vi "PS Control.vi"() -> ()   [LabVIEW 2020]
panel:
  out "Errors":T1(array[cluster]) {"Numeric 2" format="%.4f"; "Numeric" format="%.4f"}
  out "Power Supply State":T2(ring)
  out "Output Cluster":T3 {"MaxLambdaCurrent [A]" format="%.2f"; "LambdaRates [A/min]" format="%.5e"; "MaxNormalCurrent [A]" format="%.2f"; "StabilitySetting [%]" format="%.2f"; "FieldCurrentRatio [T/A]" format="%.2f"; "SwitchWaitTime [s]" format="%.2f"; "SwitchHtrCurrent [mA]" format="%.2f"; "TrainRates [A/min]" format="%.5e"; "NormalRates [A/min]" format="%.5e"; "Breakpts [A]" format="%.5e"}
  in  "Local Enable":bool
  in  "Lambda Mode":bool
  in  "Training Mode":bool
  out "Lambda":bool
  out "Train":bool
  out "Persistent Field":dbl format="%.4f"
  out "Persistence Status":string
  out "Persistent":bool
  in  "Return from persistence":bool
  in  "Make Persistent":bool
  in  "Ramp to Zero":bool
  in  "Hold":bool
  in  "Ramp to Setpoint":bool
  in  "Slew Rate [T/min]":dbl min=0.0 max=5.0 step=0.1 format="%.5f"
  in  "Setpoint [T]":dbl format="%.5f"
  out "Magnet \nVoltage":dbl format="%.2f"
  out "Field [T]":dbl format="%.4f"
  out "Switch Heater Error":bool
  out "Switch heater \nconfirmed":bool
  out "Switch Heater":bool
  in  "VISA session":refnum<visa-resource-name>="GPIB0::22::INSTR"
  in  "stop":bool
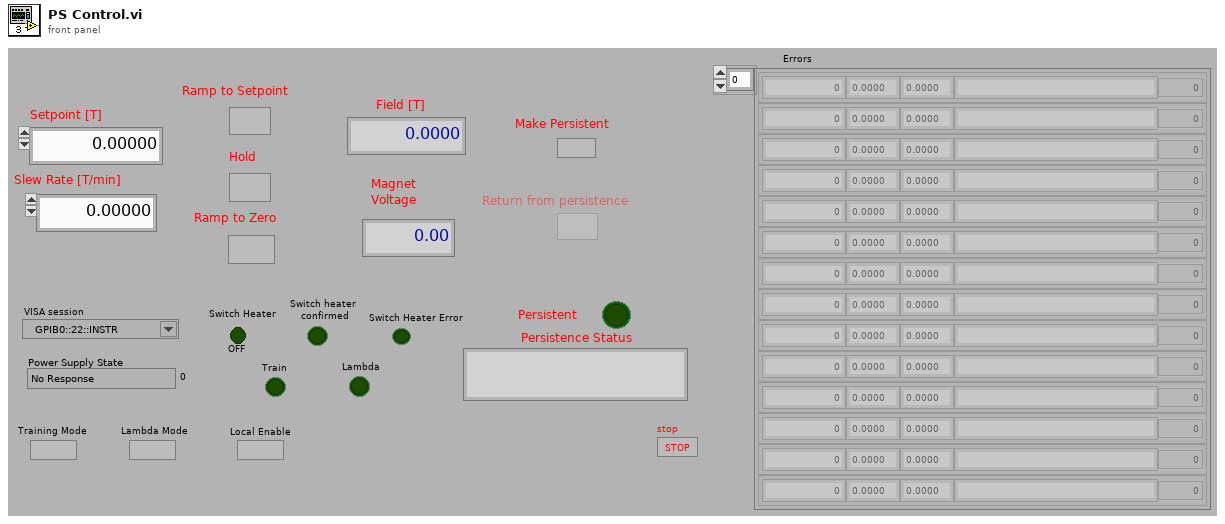
[diagram p1: front panel]
types:
  T1 = cluster{"Index 2":i32, "Numeric":dbl, "Numeric 2":dbl, "String":string, "Read ÆTime(ms)":u32}[]
  T2 = enum16{"No Response", "Ramping to programmed field ", "Holding at programmed field", "Paused", "Ramp Manual Up", "Ramp Manual Down", "Ramping to Zero", "QUENCH", "Heating Persistence Switch", "At Zero Current"}
  T3 = cluster{"Breakpts [A]":dbl[], "NormalRates [A/min]":dbl[], "TrainRates [A/min]":dbl[], "SwitchHtrCurrent [mA]":dbl, "SwitchWaitTime [s]":dbl, "FieldCurrentRatio [T/A]":dbl, "StabilitySetting [%]":dbl, "MaxNormalCurrent [A]":dbl, "Magnet ID":string, "LambdaRates [A/min]":dbl[], "MaxLambdaCurrent [A]":dbl}
  T4 = enum16{"Normal", "Train", "Lambda", "Train & Lambda"}
  T5 = enum8{"Enabled", "Disabled", "Disabled and Grayed Out"}
  T6 = cluster{i32, "Persistent Field":dbl, "Persistent Field":dbl, "String Response":string, "Read ∆ Time":dbl}
  T7 = cluster{"Index 2":i32, "Persistent Field":dbl, "Persistent Field":dbl, "String Response":string, "Read ∆ Time":dbl}[]
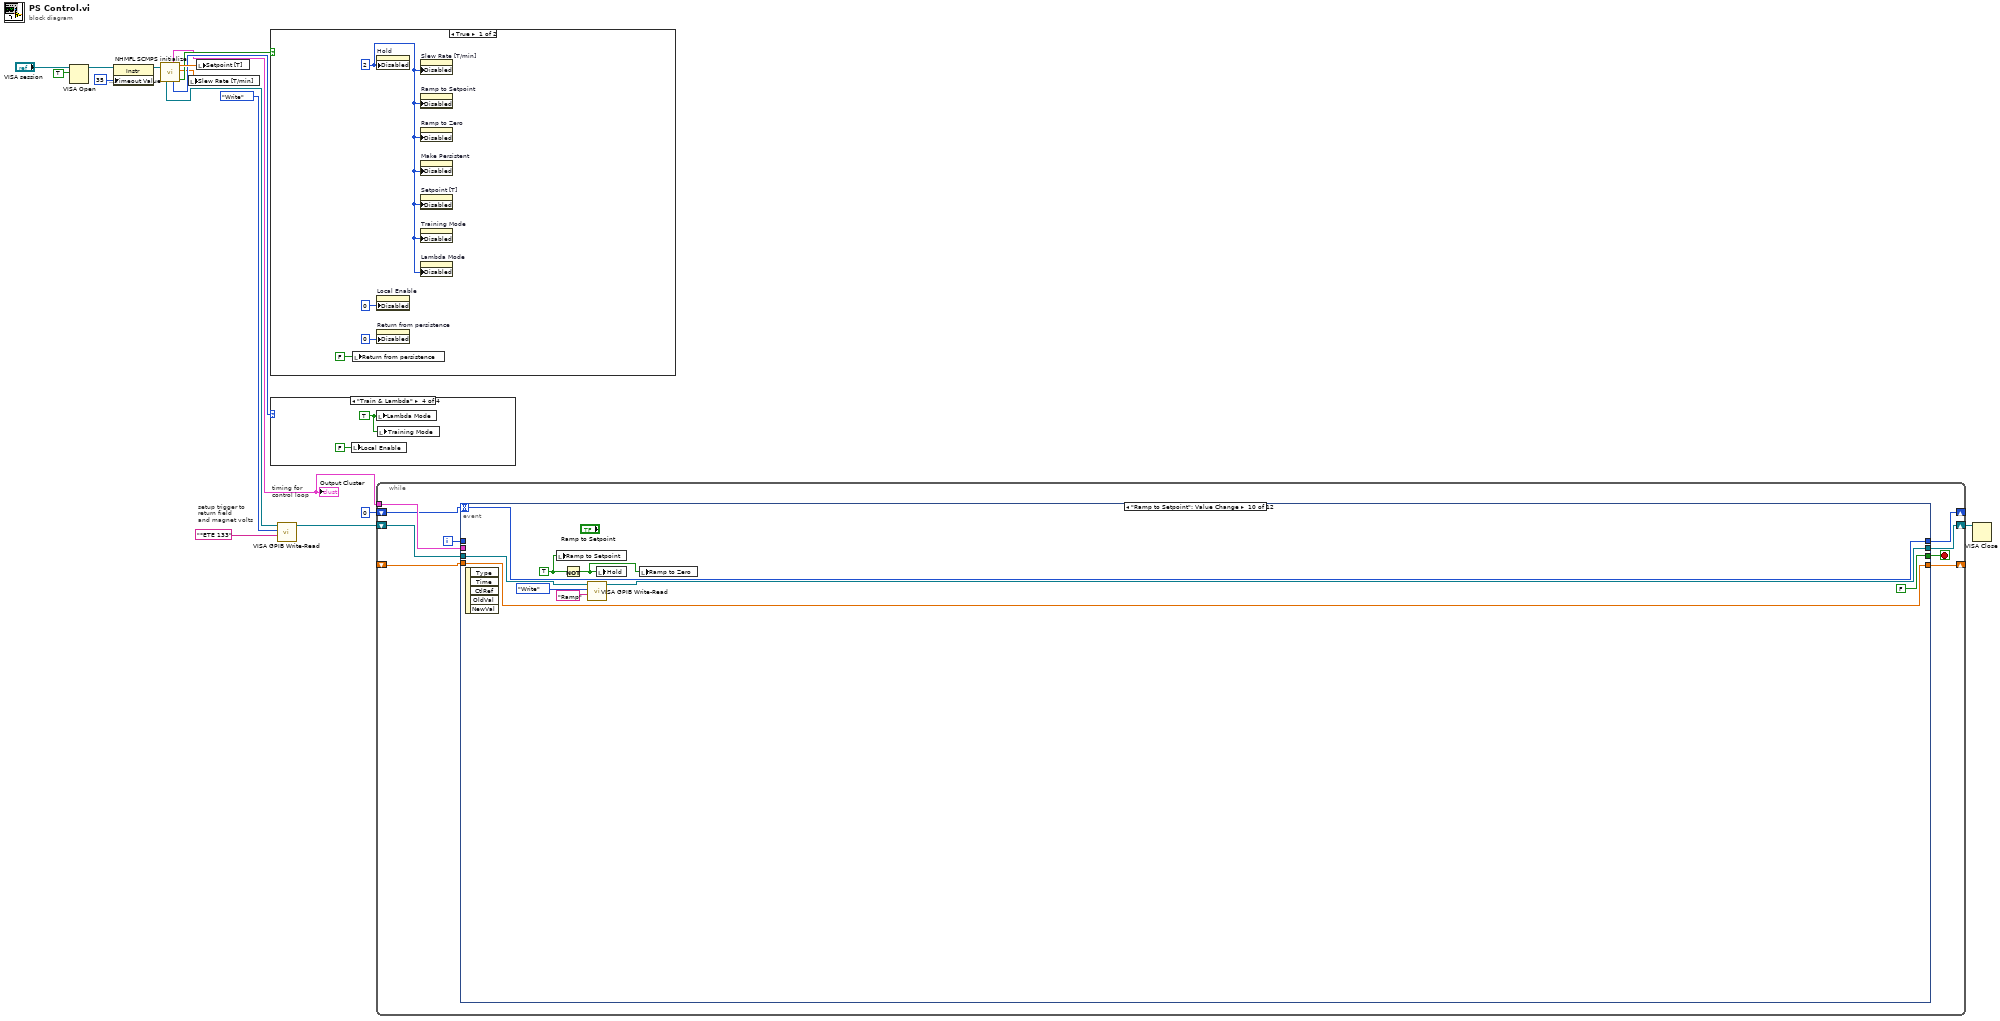
[diagram p0: block diagram]
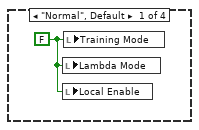
[diagram p2: hidden frame]
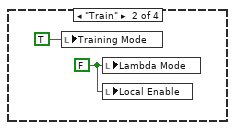
[diagram p3: hidden frame]
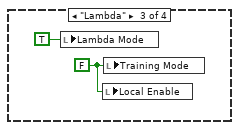
[diagram p4: hidden frame]
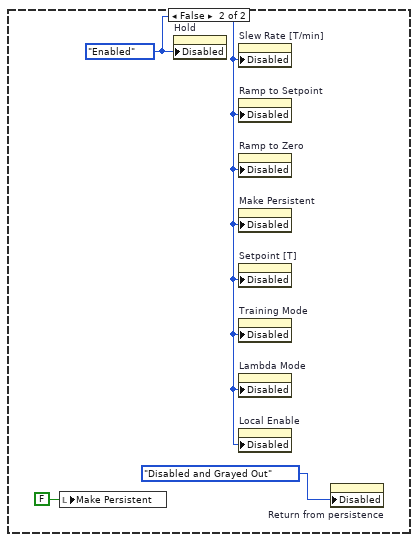
[diagram p5: hidden frame]
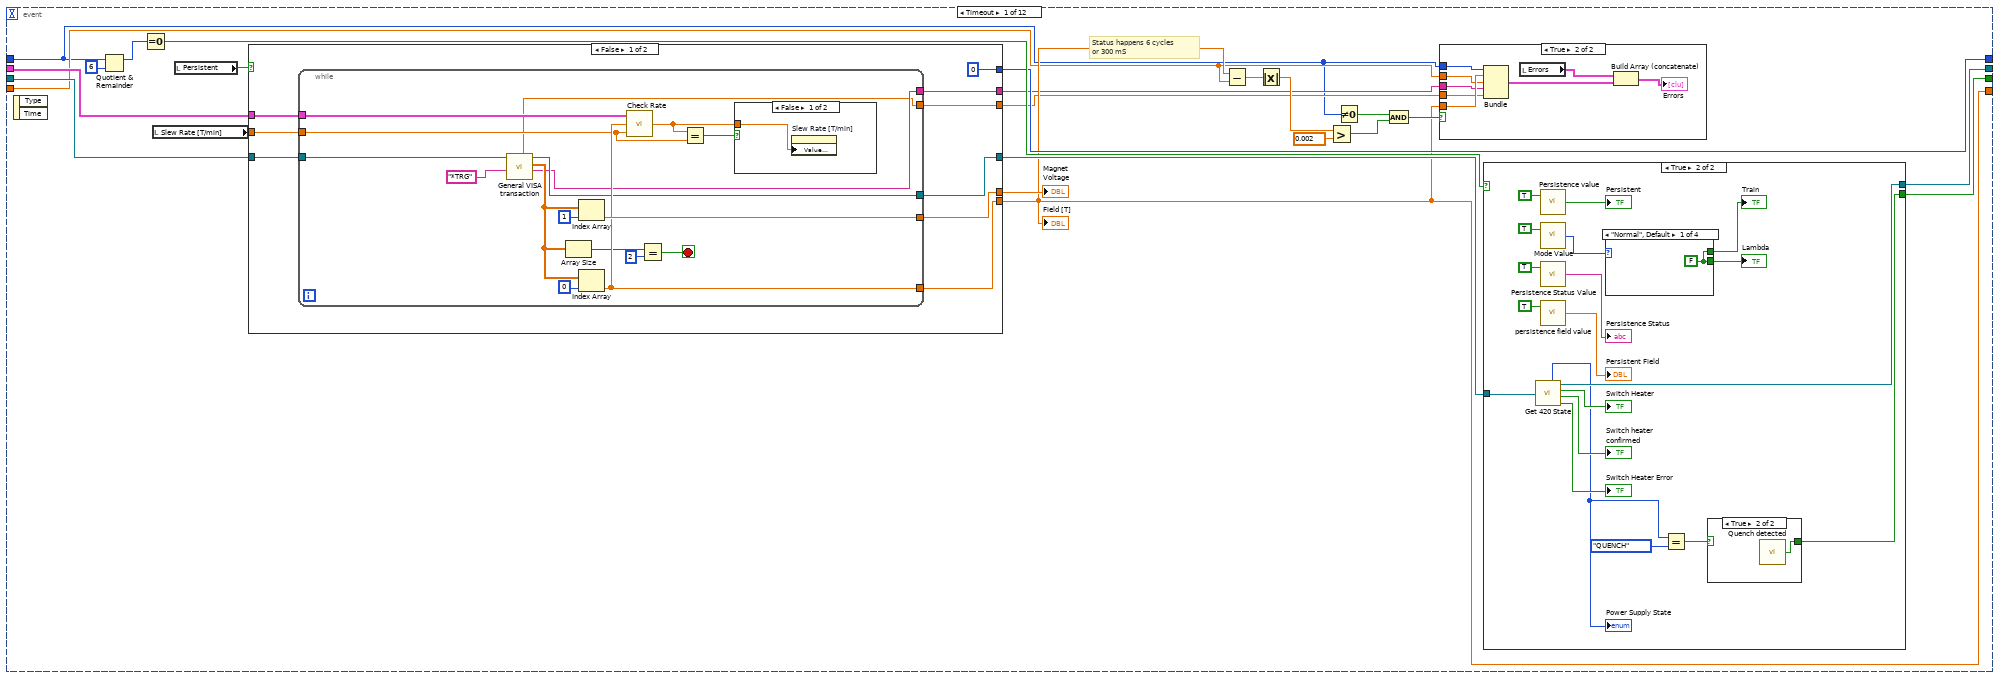
[diagram p6: hidden frame]
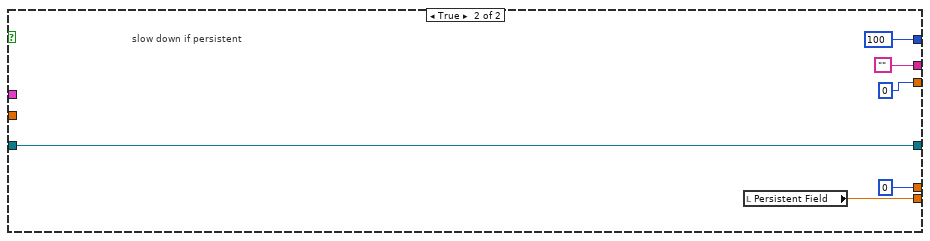
[diagram p9: hidden frame]
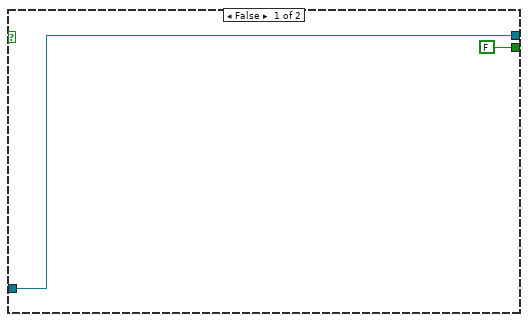
[diagram p10: hidden frame]
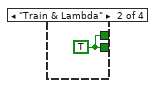
[diagram p12: hidden frame]
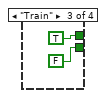
[diagram p13: hidden frame]
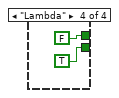
[diagram p14: hidden frame]
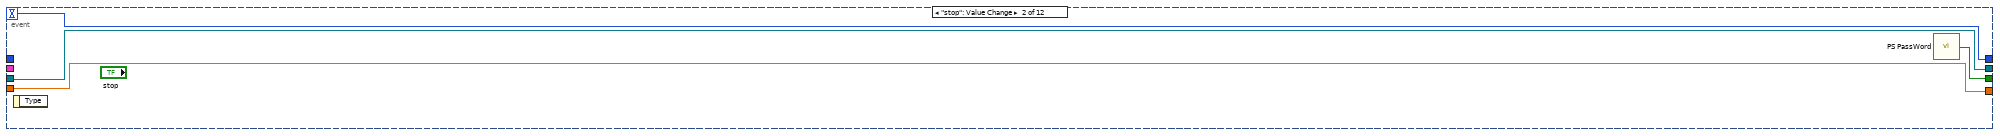
[diagram p15: hidden frame]
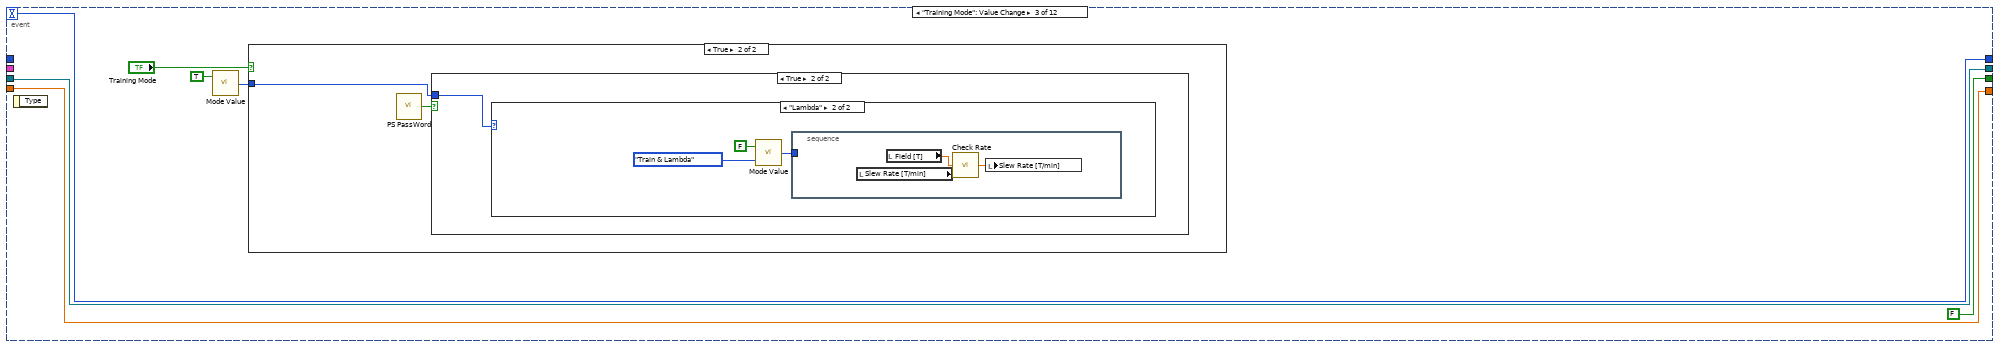
[diagram p16: hidden frame]
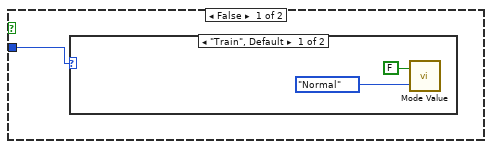
[diagram p17: hidden frame]
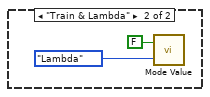
[diagram p18: hidden frame]
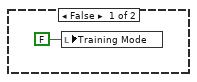
[diagram p19: hidden frame]
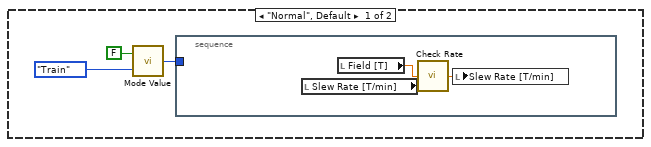
[diagram p20: hidden frame]
diagram:
  # "timing for \ncontrol loop"
  # "setup trigger to \nreturn field\nand magnet volts"
  n1 = VISA Open(duplicate session (F)=TRUE, VISA resource name="VISA session") -> (VISA resource name=w3:refnum<visa-resource-name>)  [unwired: 3 in, 1 out]
  n2 = property class="Instr"(reference=w3, "General Settings:Timeout Value"=u32 35) -> (reference out=w7:refnum<visa-resource-name>)  [unwired: 1 in, 1 out]
  n3 = call "NHMFL SCMPS initialize.vi"("VISA session"=w7) -> ("dup VISA session"=w5:refnum<visa-resource-name>, "Output Cluster"=w6:T3, "Mode Out"=w11:T4, "Programmed Field"=w14:dbl, "Ramp Rate"=w10:dbl, "Persistent"=w12:bool)  [unwired: 1 out]
  "Output Cluster" <- w6
  n4 = local write "Slew Rate [T/min]"(w10) -> ()
  n5 = local write "Setpoint [T]"(w14) -> ()
  n6 = case shown="True" w12 {
    frame True {
      w18 = 2
      n7 = local write "Return from persistence"(FALSE ("Return from persistence")) -> ()
      n8 = property on="Hold" class="Bool (strict)"("Disabled"=w18) -> ()  [unwired: 2 in, 2 out]
      n9 = property on="Local Enable" class="Bool (strict)"("Disabled"=u8 0) -> ()  [unwired: 2 in, 2 out]
      n10 = property on="Return from persistence" class="Bool (strict)"("Disabled"=u8 0) -> ()  [unwired: 2 in, 2 out]
      n11 = property on="Slew Rate [T/min]" class="DigNum (strict)"("Disabled"=w18) -> ()  [unwired: 2 in, 2 out]
      n12 = property on="Ramp to Setpoint" class="Bool (strict)"("Disabled"=w18) -> ()  [unwired: 2 in, 2 out]
      n13 = property on="Ramp to Zero" class="Bool (strict)"("Disabled"=w18) -> ()  [unwired: 2 in, 2 out]
      n14 = property on="Make Persistent" class="Bool (strict)"("Disabled"=w18) -> ()  [unwired: 2 in, 2 out]
      n15 = property on="Setpoint [T]" class="DigNum (strict)"("Disabled"=w18) -> ()  [unwired: 2 in, 2 out]
      n16 = property on="Training Mode" class="Bool (strict)"("Disabled"=w18) -> ()  [unwired: 2 in, 2 out]
      n17 = property on="Lambda Mode" class="Bool (strict)"("Disabled"=w18) -> ()  [unwired: 2 in, 2 out]
    }
    frame False {
      w22 = T5."Enabled" ("Disabled")
      n18 = local write "Make Persistent"(FALSE ("Return from persistence")) -> ()
      n19 = property on="Hold" class="Bool (strict)"("Disabled"=w22) -> ()  [unwired: 2 in, 2 out]
      n20 = property on="Slew Rate [T/min]" class="DigNum (strict)"("Disabled"=w22) -> ()  [unwired: 2 in, 2 out]
      n21 = property on="Ramp to Setpoint" class="Bool (strict)"("Disabled"=w22) -> ()  [unwired: 2 in, 2 out]
      n22 = property on="Ramp to Zero" class="Bool (strict)"("Disabled"=w22) -> ()  [unwired: 2 in, 2 out]
      n23 = property on="Make Persistent" class="Bool (strict)"("Disabled"=w22) -> ()  [unwired: 2 in, 2 out]
      n24 = property on="Setpoint [T]" class="DigNum (strict)"("Disabled"=w22) -> ()  [unwired: 2 in, 2 out]
      n25 = property on="Training Mode" class="Bool (strict)"("Disabled"=w22) -> ()  [unwired: 2 in, 2 out]
      n26 = property on="Lambda Mode" class="Bool (strict)"("Disabled"=w22) -> ()  [unwired: 2 in, 2 out]
      n27 = property on="Local Enable" class="Bool (strict)"("Disabled"=w22) -> ()  [unwired: 2 in, 2 out]
      n28 = property on="Return from persistence" class="Bool (strict)"("Disabled"=T5."Disabled and Grayed Out") -> ()  [unwired: 2 in, 2 out]
    }
  }
  n29 = case shown="\"Train & Lambda\"" w11 {
    frame "Normal", Default {
      w24 = FALSE ("Training Mode")
      n30 = local write "Lambda Mode"(w24) -> ()
      n31 = local write "Local Enable"(w24) -> ()
      n32 = local write "Training Mode"(w24) -> ()
    }
    frame "Train" {
      w26 = FALSE
      n33 = local write "Training Mode"(TRUE) -> ()
      n34 = local write "Lambda Mode"(w26) -> ()
      n35 = local write "Local Enable"(w26) -> ()
    }
    frame "Lambda" {
      w27 = FALSE
      n36 = local write "Lambda Mode"(TRUE) -> ()
      n37 = local write "Local Enable"(w27) -> ()
      n38 = local write "Training Mode"(w27) -> ()
    }
    frame "Train & Lambda" {
      w29 = TRUE
      n39 = local write "Local Enable"(FALSE) -> ()
      n40 = local write "Lambda Mode"(w29) -> ()
      n41 = local write "Training Mode"(w29) -> ()
    }
  }
  n42 = call "VISA GPIB Write-Read.vi"("Command"="*ETE 133" ("Command String"), "Action"=enum16{"Write", "Read", "Write & Read"}."Write", "VISA resource name"=w5) -> ("dup VISA Session"=w4:refnum<visa-resource-name>)  [unwired: 5 in, 3 out]
  n43 = while {
    tunnel: w6 -> [w38]
    shift-right: [w35] -> w1
    shift-left: w4 -> [w39]
    shift-right: [w33] -> _
    shift-left: 0 ("y") -> [w34]
    shift-right: [w32] -> _
    shift-left: _ -> [w31]
    i -> [w37]
    stop <- w36 stop-if-true
    n44 = event shown="[9] \"Ramp to Setpoint\": Value Change" {
      selector: _ -> [_ _ _ _ _ _ _ _ _ _ _ _]
      dyn-events: _ -> [_ _ _ _ _ _ _ _ _ _ _ _]
      timeout: w34 -> [_ w134 w138 w166 w194 w221 w274 w286 w316 w328 w337 w346]
      tunnel: w39 -> [w57 w135 w139 w167 w199 w231 w275 w291 w325 w335 w342 w351]
      tunnel: [w55 w136 FALSE ("Password Correct") FALSE ("Password Correct") FALSE ("Password Correct") FALSE ("Password Correct") FALSE ("Password Correct") FALSE ("Password Correct") FALSE ("Password Correct") FALSE ("Password Correct") FALSE ("Password Correct") FALSE ("Password Correct")] -> w36
      tunnel: w38 -> [w54 _ _ _ w198 w225 _ _ w318 _ _ _]
      tunnel: w37 -> [w40 _ _ _ _ _ _ _ _ _ _ _]
      tunnel: [w53 w135 w139 w167 w195 w222 w275 w290 w317 w329 w338 w347] -> w35
      tunnel: [w52 w134 w138 w166 w194 w221 w274 w286 w316 w328 w337 w346] -> w33
      tunnel: [w45 w133 w137 w165 w193 w220 w273 w285 w315 w327 w336 w345] -> w32
      tunnel: w31 -> [w43 w133 w137 w165 w193 w220 w273 w285 w315 w327 w336 w345]
      event Timeout {
        # "Status happens 6 cycles\nor 300 mS"
        n45 = event-data() -> ()  [unwired: 1 in, 2 out]
        n46 = Quotient & Remainder(x=w40, y=6) -> (x-y*floor(x/y)=w44:i32)  [unwired: 1 out]
        n47 = Equal To 0?(x=w44) -> (x = 0?=w61:bool)
        n48 = local read "Slew Rate [T/min]"() -> (w60:dbl)
        n49 = local read "Persistent"() -> (w59:bool)
        n50 = case shown="False" w59 {
          tunnel: w57 -> [w79 w101]
          tunnel: [w77 w103] -> w45
          tunnel: [w78 0] -> w58
          tunnel: w54 -> [w76 _]
          tunnel: w60 -> [w75 _]
          tunnel: [w74 w101] -> w56
          tunnel: [0 ("y") 100 ("y")] -> w52
          tunnel: [w72 "" ("String Response")] -> w42
          tunnel: [w71 u32 0 ("Read ÆTime")] -> w41
          frame False {
            n51 = while {
              tunnel: w79 -> [w83]
              tunnel: [w96] -> w78
              tunnel: [w95] -> w77
              tunnel: w76 -> [w94]
              tunnel: w75 -> [w86]
              tunnel: [w82] -> w74
              tunnel: [w81] -> w72
              tunnel: [w80] -> w71
              stop <- w87 stop-if-true
              n52 = call "General VISA transaction.vi"("Command String"="*TRG", "VISA Session"=w83) -> ("String Resonse"=w81:string, "Measurement"=w90:dbl[], "dup VISA Session"=w82:refnum<visa-resource-name>, "Read ∆ Time"=w80:dbl)  [unwired: 4 in, 2 out]
              n53 = Array Size(array=w90) -> (size(s)=w89:i32)
              n54 = Index Array(array=w90, index=1) -> (element=w96:dbl)
              n55 = Index Array(array=w90, index=0) -> (element=w95:dbl)
              n56 = call "Check Rate.vi"("Rate"=w86, "Field"=w95, "input cluster"=w94) -> ("Checked Rate"=w84:dbl)
              n57 = Equal?(x=w89, y=2) -> (x = y?=w87:bool)
              n58 = Equal?(x=w84, y=w86) -> (x = y?=w85:bool)
              n59 = case shown="False" w85 {
                tunnel: w84 -> [w97 _]
                frame False {
                  n60 = property on="Slew Rate [T/min]" class="DigNum (strict)"("Value (Signaling)"=w97) -> ()  [unwired: 2 in, 2 out]
                }
                frame True {
                }
              }
            }
          }
          frame True {
            # "slow down if persistent"
            n61 = local read "Persistent Field"() -> (w103:dbl)
          }
        }
        "Field [T]" <- w45
        "Magnet \nVoltage" <- w58
        n62 = Subtract(x=w45, y=w43) -> (x-y=w51:dbl)
        n63 = Absolute Value(x=w51) -> (abs(x)=w50:dbl)
        n64 = Greater?(x=w50, y=0.002) -> (0:w49:bool)
        n65 = Not Equal To 0?(x=w40) -> (x != 0?=w48:bool)
        n66 = And(x=w48, y=w49) -> (x .and. y?=w46:bool)
        n67 = case shown="True" w46 {
          tunnel: w45 -> [_ w70]
          tunnel: w43 -> [_ w69]
          tunnel: w42 -> [_ w67]
          tunnel: w40 -> [_ w64]
          tunnel: w41 -> [_ w63]
          frame False {
          }
          frame True {
            n68 = Bundle(w64, "Persistent Field"=w70, "Persistent Field"=w69, "String Response"=w67, "Read ∆ Time"=w63) -> (w66:T6)  [unwired: 1 in]
            n69 = local read "Errors"() -> (w68:T1)
            n70 = Build Array (concatenate)(w68, w66) -> (→"Errors":T7)
          }
        }
        n71 = case shown="True" w61 {
          tunnel: w56 -> [w104 w108]
          tunnel: [FALSE w109] -> w55
          tunnel: [w104 w107] -> w53
          frame False {
          }
          frame True {
            n72 = call "Get 420 State.vi"("VISA session"=w108) -> ("State"=w106:T2, "dup VISA session"=w107:refnum<visa-resource-name>, "Switch Heater"=→"Switch Heater":bool, "Switch heater \nconfirmed"=→"Switch heater \nconfirmed":bool, "Switch Heater Error"=→"Switch Heater Error":bool)  [unwired: 1 out]
            "Power Supply State" <- w106
            n73 = call "Persistence value.vi"("Read/Write this vi"=TRUE) -> ("Persistence Out"=→"Persistent":bool)  [unwired: 1 in]
            n74 = call "Mode Value.vi"("Read/Write this vi"=TRUE) -> ("Mode Out"=w120:T4)  [unwired: 1 in]
            n75 = call "Persistence Status Value.vi"("Read/Write this vi"=TRUE) -> ("Persistence Status Out"=→"Persistence Status":string)  [unwired: 1 in]
            n76 = call "persistence field value.vi"("Read/Write this vi"=TRUE) -> ("Persistent Field Out"=→"Persistent Field":dbl)  [unwired: 1 in]
            n77 = case shown="\"Normal\", Default" w120 {
              tunnel: [w127 w128 TRUE FALSE] -> w121
              tunnel: [w127 w128 FALSE TRUE] -> w122
              frame "Normal", Default {
                w127 = FALSE
              }
              frame "Train & Lambda" {
                w128 = TRUE
              }
              frame "Train" {
              }
              frame "Lambda" {
              }
            }
            "Train" <- w121
            "Lambda" <- w122
            n78 = Equal?(x=w106, y=T2."QUENCH" ("x")) -> (x = y?=w111:bool)
            n79 = case shown="True" w111 {
              selector: w111 -> [w125 _]
              tunnel: [w125 w126] -> w109
              frame False {
              }
              frame True {
                n80 = call "Quench detected.vi"() -> ("Stop"=w126:bool)
              }
            }
          }
        }
      }
      event "stop": Value Change {
        n81 = event-data() -> ()  [unwired: 1 in, 1 out]
        n82 = call "PS PassWord.vi"() -> ("Password Correct"=w136:bool)  [unwired: 2 in]
      }
      event "Training Mode": Value Change {
        n83 = event-data() -> ()  [unwired: 1 in, 1 out]
        n84 = call "Mode Value.vi"("Read/Write this vi"=TRUE) -> ("Mode Out"=w141:T4)  [unwired: 1 in]
        n85 = case shown="True" "Training Mode" {
          tunnel: w141 -> [w144 w149]
          frame False {
            n86 = case shown="\"Train\", Default" w144 {
              frame "Train", Default {
                n87 = call "Mode Value.vi"("Mode In"=T4."Normal", "Read/Write this vi"=FALSE) -> ()  [unwired: 1 out]
              }
              frame "Train & Lambda" {
                n88 = call "Mode Value.vi"("Mode In"=T4."Lambda", "Read/Write this vi"=FALSE) -> ()  [unwired: 1 out]
              }
            }
          }
          frame True {
            n89 = call "PS PassWord.vi"() -> ("Password Correct"=w150:bool)  [unwired: 2 in]
            n90 = case shown="True" w150 {
              tunnel: w149 -> [_ w152]
              frame False {
                n91 = local write "Training Mode"(FALSE ("Train")) -> ()
              }
              frame True {
                n92 = case shown="\"Lambda\"" w152 {
                  frame "Normal", Default {
                    n93 = call "Mode Value.vi"("Mode In"=T4."Train", "Read/Write this vi"=FALSE) -> ("Mode Out"=w153:T4)
                    n94 = stacked-sequence {
                      tunnel: w153 -> [_]
                      frame #0 {
                        n95 = local read "Slew Rate [T/min]"() -> (w158:dbl)
                        n96 = local read "Field [T]"() -> (w157:dbl)
                        n97 = call "Check Rate.vi"("Rate"=w158, "Field"=w157) -> ("Checked Rate"=w156:dbl)  [unwired: 1 in]
                        n98 = local write "Slew Rate [T/min]"(w156) -> ()
                      }
                    }
                  }
                  frame "Lambda" {
                    n99 = call "Mode Value.vi"("Mode In"=T4."Train & Lambda", "Read/Write this vi"=FALSE) -> ("Mode Out"=w159:T4)
                    n100 = stacked-sequence {
                      tunnel: w159 -> [_]
                      frame #0 {
                        n101 = local read "Slew Rate [T/min]"() -> (w164:dbl)
                        n102 = local read "Field [T]"() -> (w163:dbl)
                        n103 = call "Check Rate.vi"("Rate"=w164, "Field"=w163) -> ("Checked Rate"=w162:dbl)  [unwired: 1 in]
                        n104 = local write "Slew Rate [T/min]"(w162) -> ()
                      }
                    }
                  }
                }
              }
            }
          }
        }
      }
      event "Lambda Mode": Value Change {
        n105 = event-data() -> ()  [unwired: 1 in, 1 out]
        n106 = call "Mode Value.vi"("Read/Write this vi"=TRUE) -> ("Mode Out"=w169:T4)  [unwired: 1 in]
        n107 = case shown="True" "Lambda Mode" {
          tunnel: w169 -> [w172 w177]
          frame False {
            n108 = case shown="\"Lambda\", Default" w172 {
              frame "Lambda", Default {
                n109 = call "Mode Value.vi"("Mode In"=T4."Normal", "Read/Write this vi"=FALSE) -> ()  [unwired: 1 out]
              }
              frame "Train & Lambda" {
                n110 = call "Mode Value.vi"("Mode In"=T4."Train", "Read/Write this vi"=FALSE) -> ()  [unwired: 1 out]
              }
            }
          }
          frame True {
            n111 = call "PS PassWord.vi"() -> ("Password Correct"=w178:bool)  [unwired: 2 in]
            n112 = case shown="True" w178 {
              tunnel: w177 -> [_ w180]
              frame False {
                n113 = local write "Lambda Mode"(FALSE) -> ()
              }
              frame True {
                n114 = case shown="\"Train\"" w180 {
                  frame "Train" {
                    n115 = call "Mode Value.vi"("Mode In"=T4."Train & Lambda", "Read/Write this vi"=FALSE) -> ("Mode Out"=w181:T4)
                    n116 = stacked-sequence {
                      tunnel: w181 -> [_]
                      frame #0 {
                        n117 = local read "Slew Rate [T/min]"() -> (w186:dbl)
                        n118 = local read "Field [T]"() -> (w185:dbl)
                        n119 = call "Check Rate.vi"("Rate"=w186, "Field"=w185) -> ("Checked Rate"=w184:dbl)  [unwired: 1 in]
                        n120 = local write "Slew Rate [T/min]"(w184) -> ()
                      }
                    }
                  }
                  frame "Normal", Default {
                    n121 = call "Mode Value.vi"("Mode In"=T4."Lambda", "Read/Write this vi"=FALSE) -> ("Mode Out"=w187:T4)
                    n122 = stacked-sequence {
                      tunnel: w187 -> [_]
                      frame #0 {
                        n123 = local read "Slew Rate [T/min]"() -> (w192:dbl)
                        n124 = local read "Field [T]"() -> (w191:dbl)
                        n125 = call "Check Rate.vi"("Rate"=w192, "Field"=w191) -> ("Checked Rate"=w190:dbl)  [unwired: 1 in]
                        n126 = local write "Slew Rate [T/min]"(w190) -> ()
                      }
                    }
                  }
                }
              }
            }
          }
        }
      }
      event "Local Enable": Value Change {
        n127 = event-data() -> ("NewVal"=w197:bool)  [unwired: 1 in]
        n128 = case shown="True" w197 {
          tunnel: w199 -> [w202 w210]
          tunnel: w198 -> [_ w209]
          tunnel: [w200 w207] -> w195
          frame False {
            n129 = call "VISA GPIB Write-Read.vi"("Command"="SYST:REM" ("Command String"), "Action"=enum16{"Write", "Read", "Write & Read"}."Write", "VISA resource name"=w202) -> ("dup VISA Session"=w201:refnum<visa-resource-name>)  [unwired: 5 in, 3 out]
            n130 = stacked-sequence {
              tunnel: w201 -> [w205]
              tunnel: [w205] -> w200
              frame #0 {
                n131 = local write "Local Enable"(FALSE ("Local Enable")) -> ()
              }
            }
          }
          frame True {
            n132 = call "PS PassWord.vi"() -> ("Password Correct"=w208:bool)  [unwired: 2 in]
            n133 = case shown="True" w208 {
              tunnel: w210 -> [w211 w215]
              tunnel: w209 -> [_ _]
              tunnel: [w211 w213] -> w207
              frame False {
                n134 = local write "Local Enable"(FALSE) -> ()
              }
              frame True {
                n135 = call "VISA GPIB Write-Read.vi"("Command"="SYST:LOC" ("Command String"), "Action"=enum16{"Write", "Read", "Write & Read"}."Write", "VISA resource name"=w215) -> ("dup VISA Session"=w214:refnum<visa-resource-name>)  [unwired: 5 in, 3 out]
                n136 = stacked-sequence {
                  tunnel: w214 -> [w218]
                  tunnel: [w218] -> w213
                  frame #0 {
                    n137 = local write "Local Enable"(TRUE) -> ()
                  }
                }
              }
            }
          }
        }
      }
      event "Setpoint [T]": Value Change {
        n138 = event-data() -> ()  [unwired: 1 in, 5 out]
        n139 = call "Mode Value.vi"("Read/Write this vi"=TRUE) -> ("Mode Out"=w227:T4)  [unwired: 1 in]
        n140 = case shown="\"Train & Lambda\"" w227 {
          tunnel: "Setpoint [T]" -> [w235 w244 w254 w264]
          tunnel: w225 -> [w242 w252 w262 w272]
          tunnel: [w234 w246 w256 w266] -> w224
          frame "Normal", Default {
            n141 = Unbundle By Name(w242) -> ("MaxNormalCurrent [A]"=w240:dbl, "FieldCurrentRatio [T/A]"=w239:dbl)
            n142 = Multiply(x=w240, y=w239) -> (x*y=w241:dbl)
            n143 = Absolute Value(x=w235) -> (abs(x)=w238:dbl)
            n144 = In Range and Coerce(upper limit=w241, x=w238, lower limit=0.0) -> (coerced(x)=w236:dbl)  [unwired: 1 out]
            n145 = Sign(1:w235) -> (0:w233:dbl)
            n146 = Multiply(x=w236, y=w233) -> (x*y=w234:dbl)
          }
          frame "Train" {
            n147 = Unbundle By Name(w252) -> ("MaxNormalCurrent [A]"=w250:dbl, "FieldCurrentRatio [T/A]"=w249:dbl)
            n148 = Multiply(x=w250, y=w249) -> (x*y=w251:dbl)
            n149 = Absolute Value(x=w244) -> (abs(x)=w248:dbl)
            n150 = In Range and Coerce(upper limit=w251, x=w248, lower limit=0.0) -> (coerced(x)=w245:dbl)  [unwired: 1 out]
            n151 = Sign(1:w244) -> (0:w243:dbl)
            n152 = Multiply(x=w245, y=w243) -> (x*y=w246:dbl)
          }
          frame "Lambda" {
            n153 = Unbundle By Name(w262) -> ("MaxLambdaCurrent [A]"=w260:dbl, "FieldCurrentRatio [T/A]"=w259:dbl)
            n154 = Multiply(x=w260, y=w259) -> (x*y=w261:dbl)
            n155 = Absolute Value(x=w254) -> (abs(x)=w258:dbl)
            n156 = In Range and Coerce(upper limit=w261, x=w258, lower limit=0.0) -> (coerced(x)=w255:dbl)  [unwired: 1 out]
            n157 = Sign(1:w254) -> (0:w253:dbl)
            n158 = Multiply(x=w255, y=w253) -> (x*y=w256:dbl)
          }
          frame "Train & Lambda" {
            n159 = Unbundle By Name(w272) -> ("MaxLambdaCurrent [A]"=w270:dbl, "FieldCurrentRatio [T/A]"=w269:dbl)
            n160 = Multiply(x=w270, y=w269) -> (x*y=w271:dbl)
            n161 = Absolute Value(x=w264) -> (abs(x)=w268:dbl)
            n162 = In Range and Coerce(upper limit=w271, x=w268, lower limit=0.0) -> (coerced(x)=w265:dbl)  [unwired: 1 out]
            n163 = Sign(1:w264) -> (0:w263:dbl)
            n164 = Multiply(x=w265, y=w263) -> (x*y=w266:dbl)
          }
        }
        n165 = local write "Setpoint [T]"(w224) -> ()
        n166 = Format Into String(format string="CONF:FIELD:PROG %f" ("Command String"), w224) -> (resulting string=w230:string)  [unwired: 2 in, 1 out]
        n167 = call "VISA GPIB Write-Read.vi"("Command"=w230, "Action"=enum16{"Write", "Read", "Write & Read"}."Write", "VISA resource name"=w231) -> ("dup VISA Session"=w222:refnum<visa-resource-name>)  [unwired: 5 in, 3 out]
      }
      event "Make Persistent": Value Change {
        n168 = event-data() -> ()  [unwired: 1 in, 5 out]
        n169 = flat-sequence {
          tunnel: w275 -> [w278]
          tunnel: [w278] -> w276
          tunnel: w276 -> [w281]
          frame #0 {
            w280 = u8 2 ("Disabled")
            # "Disable controls"
            n170 = property on="Make Persistent" class="Bool (strict)"("Disabled"=w280) -> ()  [unwired: 2 in, 2 out]
            n171 = property on="Return from persistence" class="Bool (strict)"("Disabled"=w280) -> ()  [unwired: 2 in, 2 out]
            n172 = property on="Training Mode" class="Bool (strict)"("Disabled"=w280) -> ()  [unwired: 2 in, 2 out]
            n173 = property on="Lambda Mode" class="Bool (strict)"("Disabled"=w280) -> ()  [unwired: 2 in, 2 out]
            n174 = property on="Local Enable" class="Bool (strict)"("Disabled"=w280) -> ()  [unwired: 2 in, 2 out]
            n175 = property on="Persistence Status" class="Str"("Blinking"=TRUE) -> ()  [unwired: 2 in, 2 out]
            n176 = property on="Hold" class="Bool (strict)"("Disabled"=w280) -> ()  [unwired: 2 in, 2 out]
            n177 = property on="Slew Rate [T/min]" class="DigNum (strict)"("Disabled"=w280) -> ()  [unwired: 2 in, 2 out]
            n178 = property on="Ramp to Setpoint" class="Bool (strict)"("Disabled"=w280) -> ()  [unwired: 2 in, 2 out]
            n179 = property on="Ramp to Zero" class="Bool (strict)"("Disabled"=w280) -> ()  [unwired: 2 in, 2 out]
            n180 = property on="Setpoint [T]" class="DigNum (strict)"("Disabled"=w280) -> ()  [unwired: 2 in, 2 out]
          }
          frame #1 {
            # "make persistent routine"
            n181 = call "NML SCMPS make persistent.vi"("VISA session"=w281) -> ()  [unwired: 1 in, 3 out]
          }
          frame #2 {
            # "enable return from persistence control"
            n182 = local write "Return from persistence"(FALSE ("Return from persistence")) -> ()
            n183 = property on="Persistence Status" class="Str"("Blinking"=FALSE) -> ()  [unwired: 2 in, 2 out]
            n184 = property on="Return from persistence" class="Bool (strict)"("Disabled"=u8 0) -> ()  [unwired: 2 in, 2 out]
          }
        }
      }
      event "Return from persistence": Value Change {
        n185 = event-data() -> ()  [unwired: 1 in, 1 out]
        n186 = flat-sequence {
          tunnel: w291 -> [w294]
          tunnel: [w294] -> w289
          tunnel: w289 -> [w297]
          tunnel: [w296] -> w288
          tunnel: w288 -> [w307]
          tunnel: [w298] -> w287
          tunnel: [w310] -> w290
          tunnel: w287 -> [w310]
          frame #0 {
            w293 = T5."Disabled and Grayed Out" ("Disabled")
            # "disable both controls (others should already be disabled)"
            n187 = property on="Persistence Status" class="Str"("Blinking"=TRUE) -> ()  [unwired: 2 in, 2 out]
            n188 = property on="Make Persistent" class="Bool (strict)"("Disabled"=w293) -> ()  [unwired: 2 in, 2 out]
            n189 = property on="Return from persistence" class="Bool (strict)"("Disabled"=w293) -> ()  [unwired: 2 in, 2 out]
          }
          frame #1 {
            # "run return from persistence vi"
            n190 = call "NML SCMPS unpersistence.vi"("VISA session"=w297) -> ("dup VISA session"=w296:refnum<visa-resource-name>)  [unwired: 2 in, 2 out]
          }
          frame #2 {
            # "enable all controls except return from persistence \nand change rate back to normal"
            n191 = local read "Slew Rate [T/min]"() -> (w305:dbl)
            n192 = local read "Setpoint [T]"() -> (w300:dbl)
            n193 = Format Into String(format string="CONF:RAMP:RATE:FIELD %f" ("Command String"), w305) -> (resulting string=w304:string)  [unwired: 2 in, 1 out]
            n194 = call "VISA GPIB Write-Read.vi"("Command"=w304, "Action"=enum16{"Write", "Read", "Write & Read"}."Write", "VISA resource name"=w307) -> ("dup VISA Session"=w299:refnum<visa-resource-name>)  [unwired: 5 in, 3 out]
            n195 = Format Into String(format string="CONF:FIELD:PROG %f" ("Command String"), w300) -> (resulting string=w301:string)  [unwired: 2 in, 1 out]
            n196 = call "VISA GPIB Write-Read.vi"("Command"=w301, "Action"=enum16{"Write", "Read", "Write & Read"}."Write", "VISA resource name"=w299) -> ("dup VISA Session"=w298:refnum<visa-resource-name>)  [unwired: 5 in, 3 out]
          }
          frame #3 {
            w309 = T5."Enabled" ("Disabled")
            w313 = TRUE
            w314 = FALSE  # Return from persistence
            # "Return from persistence"
            n197 = local write "Hold"(w313) -> ()
            n198 = property on="Persistence Status" class="Str"("Blinking"=FALSE) -> ()  [unwired: 2 in, 2 out]
            n199 = Not(x=w313) -> (.not. x?=w312:bool)
            n200 = local write "Ramp to Setpoint"(w312) -> ()
            n201 = local write "Ramp to Zero"(w312) -> ()
            n202 = local write "Make Persistent"(w314) -> ()
            n203 = property on="Ramp to Zero" class="Bool (strict)"("Disabled"=w309) -> ()  [unwired: 2 in, 2 out]
            n204 = property on="Ramp to Setpoint" class="Bool (strict)"("Disabled"=w309) -> ()  [unwired: 2 in, 2 out]
            n205 = property on="Setpoint [T]" class="DigNum (strict)"("Disabled"=w309) -> ()  [unwired: 2 in, 2 out]
            n206 = property on="Slew Rate [T/min]" class="DigNum (strict)"("Disabled"=w309) -> ()  [unwired: 2 in, 2 out]
            n207 = property on="Hold" class="Bool (strict)"("Disabled"=w309) -> ()  [unwired: 2 in, 2 out]
            n208 = property on="Lambda Mode" class="Bool (strict)"("Disabled"=w309) -> ()  [unwired: 2 in, 2 out]
            n209 = property on="Training Mode" class="Bool (strict)"("Disabled"=w309) -> ()  [unwired: 2 in, 2 out]
            n210 = property on="Local Enable" class="Bool (strict)"("Disabled"=w309) -> ()  [unwired: 2 in, 2 out]
            n211 = property on="Make Persistent" class="Bool (strict)"("Disabled"=w309) -> ()  [unwired: 2 in, 2 out]
          }
        }
      }
      event "Slew Rate [T/min]": Value Change {
        n212 = event-data() -> ()  [unwired: 1 in, 5 out]
        n213 = local read "Field [T]"() -> (w322:dbl)
        n214 = call "Check Rate.vi"("Rate"="Slew Rate [T/min]", "Field"=w322, "input cluster"=w318) -> ("Checked Rate"=w320:dbl)
        n215 = local write "Slew Rate [T/min]"(w320) -> ()
        n216 = Format Into String(format string="CONF:RAMP:RATE:FIELD %f" ("Command String"), w320) -> (resulting string=w324:string)  [unwired: 2 in, 1 out]
        n217 = call "VISA GPIB Write-Read.vi"("Command"=w324, "Action"=enum16{"Write", "Read", "Write & Read"}."Write", "VISA resource name"=w325) -> ("dup VISA Session"=w317:refnum<visa-resource-name>)  [unwired: 5 in, 3 out]
      }
      event "Ramp to Setpoint": Value Change {
        w331 = TRUE
        n218 = event-data() -> ()  [unwired: 1 in, 5 out]
        n219 = local write "Ramp to Setpoint"(w331) -> ()
        n220 = Not(x=w331) -> (.not. x?=w332:bool)
        n221 = call "VISA GPIB Write-Read.vi"("Command"="Ramp" ("Command String"), "Action"=enum16{"Write", "Read", "Write & Read"}."Write", "VISA resource name"=w335) -> ("dup VISA Session"=w329:refnum<visa-resource-name>)  [unwired: 5 in, 3 out]
        n222 = local write "Hold"(w332) -> ()
        n223 = local write "Ramp to Zero"(w332) -> ()
      }
      event "Hold": Value Change {
        w340 = TRUE
        n224 = event-data() -> ()  [unwired: 1 in, 1 out]
        n225 = local write "Hold"(w340) -> ()
        n226 = call "VISA GPIB Write-Read.vi"("Command"="PAUSE" ("Command String"), "Action"=enum16{"Write", "Read", "Write & Read"}."Write", "VISA resource name"=w342) -> ("dup VISA Session"=w338:refnum<visa-resource-name>)  [unwired: 5 in, 3 out]
        n227 = Not(x=w340) -> (.not. x?=w341:bool)
        n228 = local write "Ramp to Setpoint"(w341) -> ()
        n229 = local write "Ramp to Zero"(w341) -> ()
      }
      event "Ramp to Zero": Value Change {
        w349 = TRUE
        n230 = event-data() -> ()  [unwired: 1 in, 5 out]
        n231 = local write "Ramp to Zero"(w349) -> ()
        n232 = Not(x=w349) -> (.not. x?=w350:bool)
        n233 = call "VISA GPIB Write-Read.vi"("Command"="ZERO" ("Command String"), "Action"=enum16{"Write", "Read", "Write & Read"}."Write", "VISA resource name"=w351) -> ("dup VISA Session"=w347:refnum<visa-resource-name>)  [unwired: 5 in, 3 out]
        n234 = local write "Hold"(w350) -> ()
        n235 = local write "Ramp to Setpoint"(w350) -> ()
      }
    }
  }
  n236 = VISA Close(VISA resource name=w1) -> ()  [unwired: 1 in, 1 out]
